vi "Read Config.vi"(8 "error in (no error)":errorcluster, 10 "Resource In":variant, 11 "Target Point in":refnum<class "Target Point.lvclass">) -> (0 "error out":errorcluster, 2 "Resource Out":variant, 3 "Target Point out":refnum<class "Target Point.lvclass">)   [LabVIEW 2020, in "Target Point.lvclass"]
uses:
  Target Point.lvclass
  C:/POLARIS Programme/POLARIS-AS-3-Cams/Submodules/HIJ Vision/Analyze/Analyze Parameter/Analyze Parameter Base/Analyze Parameter Base.lvclass
  <vilib>/Utility/config.llb/Config Data RefNum.ctl
  Target Point.lvclass/Target Point.ctl
  <vilib>/Utility/config.llb/Read Key (I32).vi
  <vilib>/Utility/config.llb/NI_LVConfig.lvlib
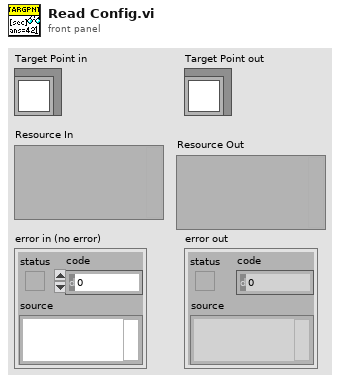
[diagram p1: front panel]
types:
  T1 = typedef "NI_LVConfig.lvlib/Config Data RefNum.ctl" = refnum<k1>
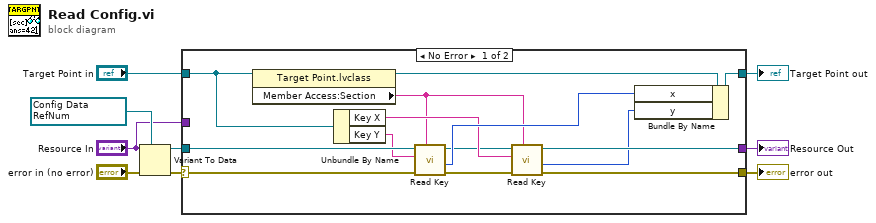
[diagram p0: block diagram]
diagram:
  w7 = T1 refnum items=["config data"] ("refnum")
  n1 = Variant To Data(error in="error in (no error)", type=w7, Variant="Resource In") -> (data=w9:T1, error out=w8:errorcluster)
  n2 = case shown="No Error" w8 {
    selector: w8 -> [w17 w25]
    tunnel: w9 -> [w23 _]
    tunnel: "Target Point in" -> [w18 w24]
    tunnel: [w21 w24] -> w4
    tunnel: [w13 w26] -> w3
    tunnel: [w11 w25] -> w2
    tunnel: "Resource In" -> [_ w26]
    frame No Error {
      n3 = property class="Target Point.lvclass"(reference=w18) -> (reference out=w19:refnum<class "Target Point.lvclass">, "Member Access:Section"=w15:string)  [unwired: 1 in, 1 out]
      n4 = Unbundle By Name(w18) -> ("Key X"=w16:string, "Key Y"=w20:string)
      n5 = call-poly <vilib>:"Read Key.vi"("section"=w15, "error in (no error)"=w17, "key"=w20, "refnum"=w23) -> ("error out"=w12:errorcluster, "value"=w22:i32, "refnum out"=w14:T1)  [unwired: 4 in, 1 out]
      n6 = call-poly <vilib>:"Read Key.vi"("section"=w15, "error in (no error)"=w12, "key"=w16, "refnum"=w14) -> ("error out"=w11:errorcluster, "value"=w10:i32, "refnum out"=w13:T1)  [unwired: 4 in, 1 out]
      n7 = Bundle By Name(cluster=w19, "x"=w22, "y"=w10) -> (w21:refnum<class "Target Point.lvclass">)
    }
    frame Error {
    }
  }
  "error out" <- w2
  "Target Point out" <- w4
  "Resource Out" <- w3
